vi "Shutdown.vi"(8 "error in (no error)":errorcluster, 11 "Transceiver Thread in":refnum<class "Transceiver Thread.lvclass">) -> (0 "error out":errorcluster, 3 "Transceiver Thread out":refnum<class "Transceiver Thread.lvclass">)   [LabVIEW 2017, in "Data Sharing Framework Core.lvlib" / "Data Sharing Framework Engine.lvlib" / "Transceiver Thread.lvclass"]
uses:
  Transceiver Thread.lvclass
  Interfaces/Transceiver Interface/Response Data.ctl
  Interfaces/Transceiver Interface/Response.ctl
  Interfaces/Transceiver Interface/Response Parameters.ctl
  Interfaces/Transceiver Interface/Transceiver Interface.lvclass
  Transceiver/Transceiver.lvclass
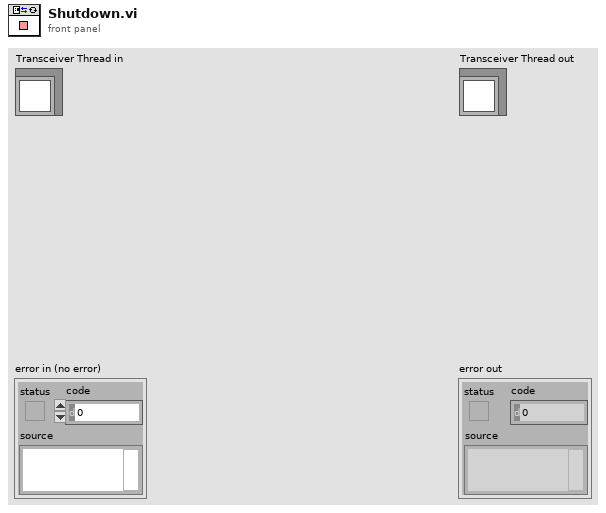
[diagram p1: front panel]
types:
  T1 = typedef "Data Sharing Framework Core.lvlib/Data Sharing Framework Engine.lvlib/Transceiver Interface.lvclass/Response Data.ctl" = cluster{"Response":T2, "Response Parameters":T3}
  T2 = typedef "Data Sharing Framework Core.lvlib/Data Sharing Framework Engine.lvlib/Transceiver Interface.lvclass/Response.ctl" = enum8{"General Ack", "Shutting Down"}
  T3 = typedef "Data Sharing Framework Core.lvlib/Data Sharing Framework Engine.lvlib/Transceiver Interface.lvclass/Response Parameters.ctl" = cluster{"arg1":u64, "arg2":u64}
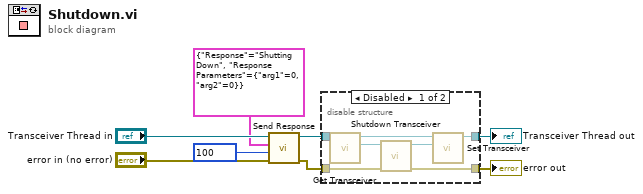
[diagram p0: block diagram]
diagram:
  n1 = call "Send Response.vi"("error in (no error)"="error in (no error)", "timeout in ms (0)"=100, "response"=T1 {"Response"=enum."Shutting Down", "Response Parameters"={"arg1"=0, "arg2"=0}}, "Transceiver Thread in"="Transceiver Thread in") -> ("error out"=w4:errorcluster, "Transceiver Thread out"=w3:refnum<class "Transceiver Thread.lvclass">)  [unwired: 5 in, 1 out]
  n2 = disable-structure shown="Disabled" {
    disable-tunnel: [w12 w17] -> w8
    disable-tunnel: [w11 w16] -> w7
    disable-tunnel: w4 -> [w10 w16]
    disable-tunnel: w3 -> [w9 w17]
    frame Disabled {
      n3 = call "Get Transceiver.vi"("Transceiver Thread in"=w9) -> ("Transceiver"=w15:refnum<class "Transceiver.lvclass">, "Transceiver Thread out"=w13:refnum<class "Transceiver Thread.lvclass">)  [unwired: 9 in]
      n4 = call-dynamic "Shutdown Transceiver.vi"("error in (no error)"=w10, "Transceiver in"=w15) -> ("error out"=w11:errorcluster, "Transceiver out"=w14:refnum<class "Transceiver.lvclass">)  [unwired: 8 in]
      n5 = call "Set Transceiver.vi"("Transceiver"=w14, "Transceiver Thread in"=w13) -> ("Transceiver Thread out"=w12:refnum<class "Transceiver Thread.lvclass">)  [unwired: 9 in]
    }
    frame Enabled {
    }
  }
  "error out" <- w7
  "Transceiver Thread out" <- w8
